vi "Test.vi"() -> ()   [LabVIEW 2015]
panel:
  in  "script path":string="C:\\Users\\tilin\\Desktop\\Vision_20160307\\Data\\CCC"
  in  "stop":bool
  in  "Run":bool
  out "data string":string
  # "<- Run之前要改"
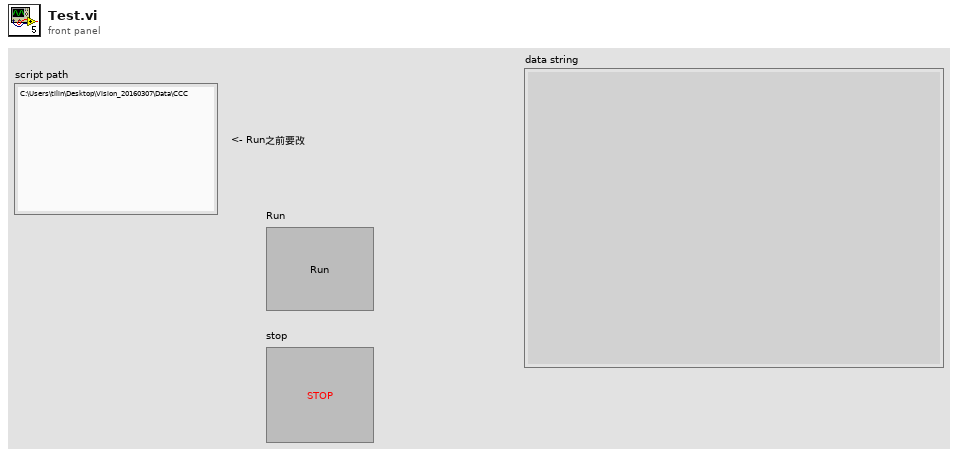
[diagram p1: front panel]
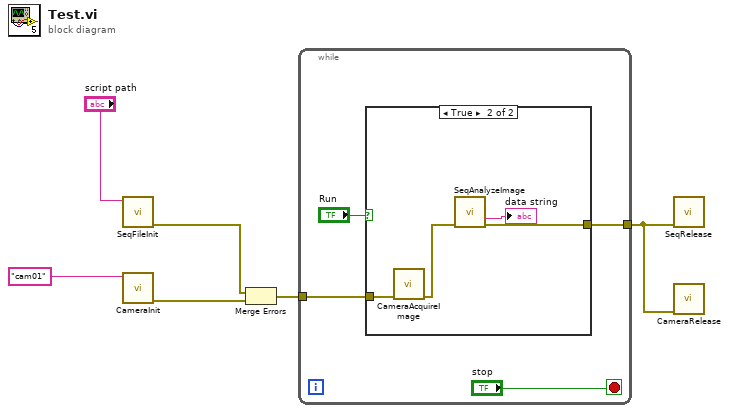
[diagram p0: block diagram]
diagram:
  n1 = call "SeqFileInit.vi"("script path"="script path") -> ("error out"=w2:errorcluster)  [unwired: 9 in, 1 out]
  n2 = call "CameraInit.vi"("CameraName"="cam01") -> ("error out"=w5:errorcluster)  [unwired: 9 in, 1 out]
  n3 = Merge Errors(w2, w5) -> (w4:errorcluster)
  n4 = while {
    tunnel: w4 -> [w9]
    tunnel: [w8] -> w1
    stop <- "stop" stop-if-true
    n5 = case shown="True" "Run" {
      tunnel: w9 -> [w11 w15]
      tunnel: [w11 w13] -> w8
      frame False {
      }
      frame True {
        n6 = call "CameraAcquireImage.vi"("error in"=w15) -> ("error out"=w14:errorcluster)  [unwired: 9 in, 1 out]
        n7 = call "SeqAnalyzeImage.vi"("error in"=w14) -> ("data string"=→"data string":string, "error out"=w13:errorcluster)  [unwired: 9 in, 4 out]
      }
    }
  }
  n8 = call "SeqRelease.vi"("error in"=w1) -> ()  [unwired: 9 in, 2 out]
  n9 = call "CameraRelease.vi"("error in"=w1) -> ()  [unwired: 9 in, 2 out]
